vi "Write Cleanup TS.vi"(8 "error in (no error)":errorcluster, 10 "Cleanup":i64, 11 "CIFCorePlugin in":refnum<class "CIFCorePlugin.lvclass">) -> (0 "error out":errorcluster, 3 "CIFCorePlugin out":refnum<class "CIFCorePlugin.lvclass">)   [LabVIEW 2021, in "CIFCorePlugin.lvclass"]
doc: "Update the timestamp. Time is U64, absolute time in nS in the appropriate clockID configured for the plugin. If a 0 is wired it will automatically get the current time."
uses:
  CIFCorePlugin.lvclass
  CIFCorePlugin.lvclass/CIFCorePlugin.ctl
  CIFUtilities/CIFLogs/Typedef/Plugin State Commands.ctl
  <vilib>/CIF Foundation/CIF Utilities/Time/System Time/LabVIEW Time to TAI Time.vi
  CIFUtilities/CIFLogs/CIFLogs.lvlib
  <vilib>/CIF Foundation/CIF Utilities/Time/Time_CIF_U.lvlib
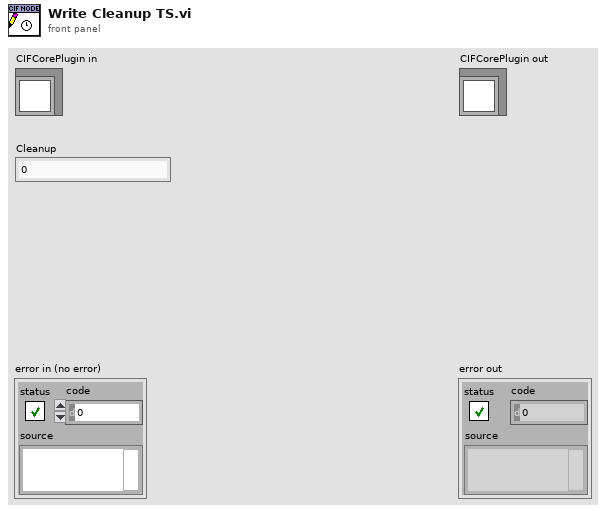
[diagram p1: front panel]
types:
  T1 = typedef "CIFLogs.lvlib/Plugin State Commands.ctl" = enum16{"Create", "Configure", "Run", "Pause", "Destroy", "Connect", "Force", "FIFO Instance"}
  T2 = typedef "CIFCorePlugin.lvclass/Energized States.ctl" = enum16{"Listen", "Prepare", "Execute", "Housekeep", "Cleanup", "Destroy"}
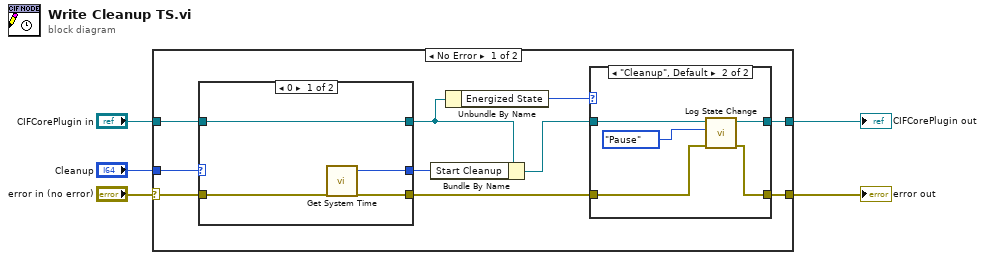
[diagram p0: block diagram]
diagram:
  n1 = case shown="No Error" "error in (no error)" {
    selector: "error in (no error)" -> [w14 w29]
    tunnel: [w8 w29] -> w4
    tunnel: [w9 w30] -> w2
    tunnel: "CIFCorePlugin in" -> [w13 w30]
    tunnel: "Cleanup" -> [w15 _]
    frame No Error {
      n2 = case shown="0" w15 {
        selector: w15 -> [_ w27]
        tunnel: w14 -> [w23 w26]
        tunnel: w13 -> [w25 w28]
        tunnel: [w25 w28] -> w7
        tunnel: [w24 w27] -> w12
        tunnel: [w23 w26] -> w10
        frame 0 {
          n3 = call <vilib>:"Get System Time.vi"() -> ("Time (ns)"=w24:i64)  [unwired: 5 in]
        }
        frame 1, Default {
        }
      }
      n4 = Bundle By Name(cluster=w7, "Start Cleanup"=w12) -> (w11:refnum<class "CIFCorePlugin.lvclass">)
      n5 = Unbundle By Name(w7) -> ("Energized State"=w6:T2)
      n6 = case shown="\"Cleanup\", Default" w6 {
        tunnel: w11 -> [w17 w22]
        tunnel: w10 -> [w16 w21]
        tunnel: [w17 w20] -> w9
        tunnel: [w16 w18] -> w8
        frame "Destroy" {
        }
        frame "Cleanup", Default {
          n7 = call "Log State Change.vi"("error in (no error)"=w21, "Command"=Plugin_State_Commands."Pause", "CIFCorePlugin in"=w22) -> ("error out"=w18:errorcluster, "CIFCorePlugin out"=w20:refnum<class "CIFCorePlugin.lvclass">)  [unwired: 7 in]
        }
      }
    }
    frame Error {
    }
  }
  "error out" <- w4
  "CIFCorePlugin out" <- w2
